vi "CTRE_Phoenix_MotorControl_ConfigClosedLoopConstants.vi"(0 "CAN Talon SRX Ref":T1={"DeviceStatus"={"status"=FALSE, "code"=0, "source"=""}, "Type"=enum."PWM", "PWM"={"PWM Channel"=enum."PWM 1", "DeadBand"={"Name"="", "maxPositivePwm"=0, "minPositivePwm"=0, "centerPwm"=0, "maxNegativePwm"=0, "minNegativePwm"=0, "angularRange"=0}}, "CAN"={"Device Number"=0, "SetOutput VI Ref"=variant(enum8{"Percent VBus", "Current", "Speed", "Position", "Voltage"} enum."Percent VBus"), "GetOutput VI Ref"=variant(refnum<k1> refnum), "Enable VI Ref"=variant(dbl 12.0), "Disable VI Ref"=variant(enum8{"Percent VBus", "Speed", "Position", "Slave", "Unchanged / Invalid", "Voltage Compensation", "Current", "Motion Profile"} enum."Percent VBus"), "Data"=variant}, "Invert"=FALSE}, 1 "slotIdx":i32, 5 "P":sgl, 7 "I":sgl, 9 "D":sgl, 11 "error in (no error)":errorcluster, 12 "F":sgl, 13 "I Zone":sgl, 14 "timeoutMs":i32) -> (4 "CAN Talon SRX Ref":T1={"DeviceStatus"={"status"=FALSE, "code"=0, "source"=""}, "Type"=enum."PWM", "PWM"={"PWM Channel"=enum."PWM 1", "DeadBand"={"Name"="", "maxPositivePwm"=0, "minPositivePwm"=0, "centerPwm"=0, "maxNegativePwm"=0, "minNegativePwm"=0, "angularRange"=0}}, "CAN"={"Device Number"=0, "SetOutput VI Ref"=variant(enum8{"Percent VBus", "Current", "Speed", "Position", "Voltage"} enum."Percent VBus"), "GetOutput VI Ref"=variant(refnum<k1> refnum), "Enable VI Ref"=variant(dbl 12.0), "Disable VI Ref"=variant(enum8{"Percent VBus", "Speed", "Position", "Slave", "Unchanged / Invalid", "Voltage Compensation", "Current", "Motion Profile"} enum."Percent VBus"), "Data"=variant}, "Invert"=FALSE}, 15 "error out":errorcluster)   [LabVIEW 2016]
doc: "Configures the closed-loop constant values."
uses:
  <vilib>/Rock Robotics/WPI/MotorControl/WPI_MotorControlDeviceRef.ctl
  <vilib>/Rock Robotics/WPI/MotorControl/WPI_MotorControlType.ctl
  <vilib>/Rock Robotics/SystemInterfaces/DIO/FPGA_DIOPWMChannel.ctl
  <vilib>/Rock Robotics/WPI/PWM/WPI_PWMDeadband.ctl
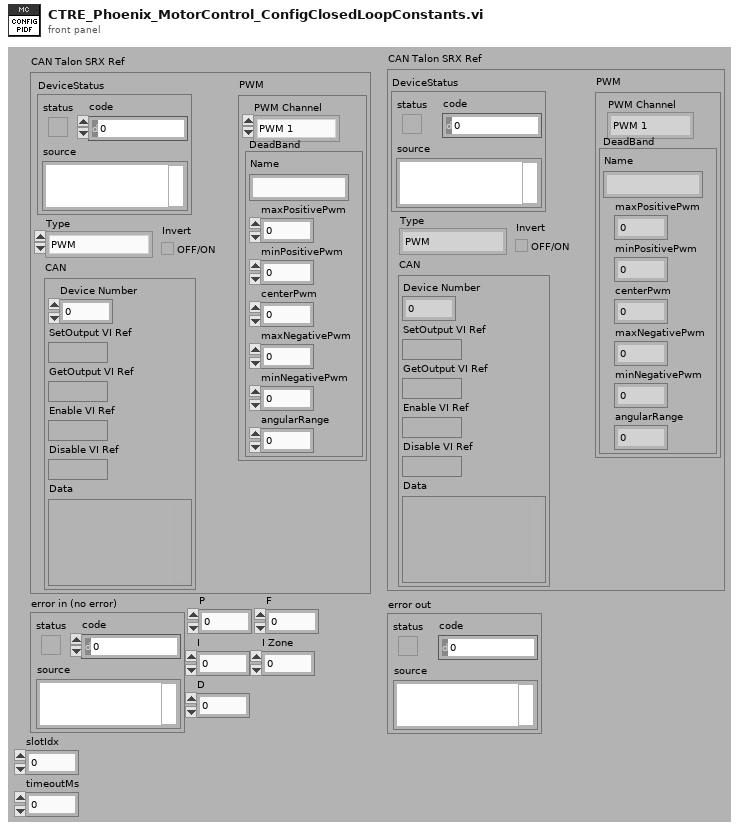
[diagram p1: front panel]
types:
  T1 = typedef "WPI_MotorControlDeviceRef.ctl" = cluster{"DeviceStatus":errorcluster, "Type":T2, "PWM":cluster{"PWM Channel":T3, "DeadBand":T4}, "CAN":cluster{"Device Number":u8, "SetOutput VI Ref":variant, "GetOutput VI Ref":variant, "Enable VI Ref":variant, "Disable VI Ref":variant, "Data":variant}, "Invert":bool}
  T2 = typedef "WPI_MotorControlType.ctl" = enum16{"PWM", "CAN"}
  T3 = typedef "FPGA_DIOPWMChannel.ctl" = enum8{"PWM 0", "PWM 1", "PWM 2", "PWM 3", "PWM 4", "PWM 5", "PWM 6", "PWM 7", "PWM 8", "PWM 9", "PWM MXP 0", "PWM MXP 1", "PWM MXP 2", "PWM MXP 3", "PWM MXP 4", "PWM MXP 5", "PWM MXP 6", "PWM MXP 7", "PWM MXP 8", "PWM MXP 9", "Invalid"}
  T4 = typedef "WPI_PWMDeadband.ctl" = cluster{"Name":string, "maxPositivePwm":i32, "minPositivePwm":i32, "centerPwm":i32, "maxNegativePwm":i32, "minNegativePwm":i32, "angularRange":u16}
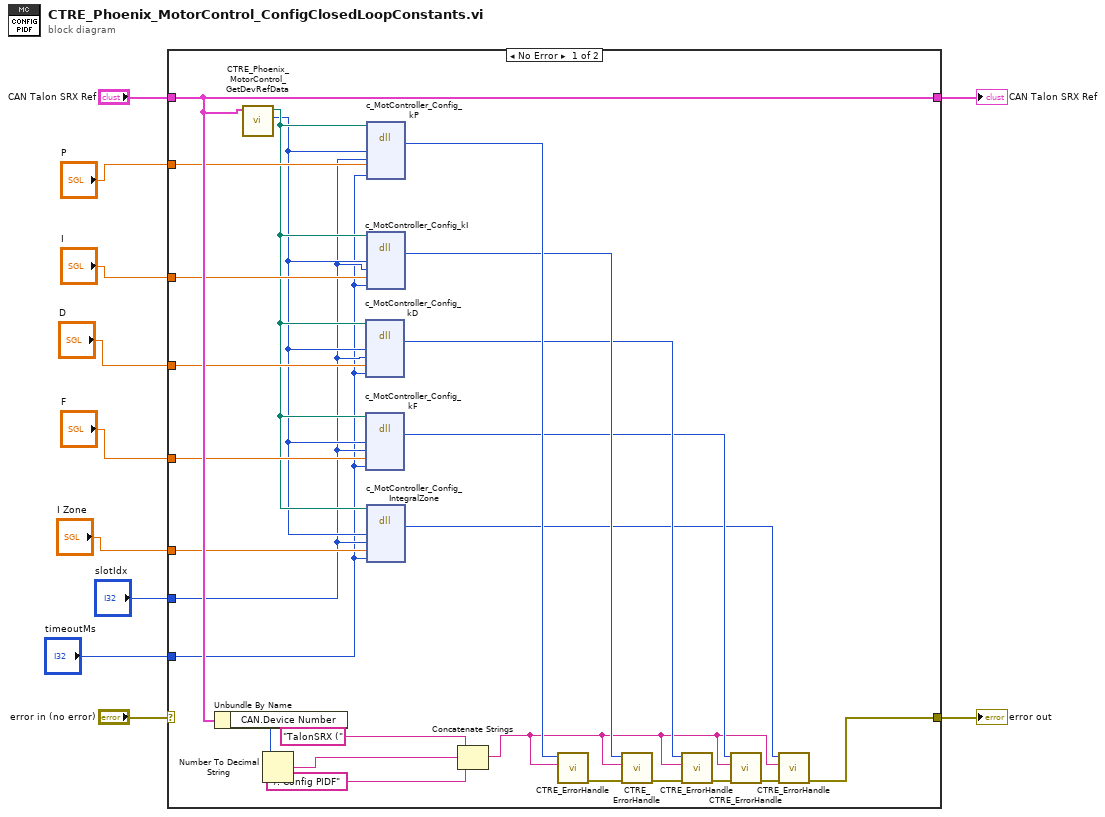
[diagram p0: block diagram]
diagram:
  n1 = case shown="No Error" "error in (no error)" {
    selector: "error in (no error)" -> [_ w38]
    tunnel: [w14 w38] -> w11
    tunnel: "CAN Talon SRX Ref" -> [w32 w37]
    tunnel: [w32 w37] -> w9
    tunnel: "P" -> [w29 _]
    tunnel: "I" -> [w28 _]
    tunnel: "D" -> [w27 _]
    tunnel: "F" -> [w26 _]
    tunnel: "I Zone" -> [w25 _]
    tunnel: "slotIdx" -> [w13 _]
    tunnel: "timeoutMs" -> [w12 _]
    frame No Error {
      n2 = Unbundle By Name(w32) -> ("CAN.Device Number"=w33:u8)
      n3 = call "CTRE_Phoenix_MotorControl_GetDevRefData.vi"("MotorControlDevRef"=w32) -> ("handle"=w23:u64, "Library"=w24:path)  [unwired: 4 in, 5 out]
      n4 = Number To Decimal String(number=w33) -> (decimal integer string=w35:string)  [unwired: 1 in]
      n5 = dll-call lib="?" fn="c_MotController_Config_kD"(path in=w24, "handle"=w23, "slotIdx"=w13, "value"=w27, "timeoutMs"=w12) -> ("ErrorCode"=w20:i32)  [unwired: 6 in, 2 out]
      n6 = dll-call lib="?" fn="c_MotController_Config_kF"(path in=w24, "handle"=w23, "slotIdx"=w13, "value"=w26, "timeoutMs"=w12) -> ("ErrorCode"=w18:i32)  [unwired: 6 in, 2 out]
      n7 = dll-call lib="?" fn="c_MotController_Config_kP"(path in=w24, "handle"=w23, "slotIdx"=w13, "value"=w29, "timeoutMs"=w12) -> ("ErrorCode"=w31:i32)  [unwired: 6 in, 2 out]
      n8 = dll-call lib="?" fn="c_MotController_Config_kI"(path in=w24, "handle"=w23, "slotIdx"=w13, "value"=w28, "timeoutMs"=w12) -> ("ErrorCode"=w22:i32)  [unwired: 6 in, 2 out]
      n9 = dll-call lib="?" fn="c_MotController_Config_IntegralZone"(path in=w24, "handle"=w23, "slotIdx"=w13, "value"=w25, "timeoutMs"=w12) -> ("ErrorCode"=w15:i32)  [unwired: 6 in, 2 out]
      n10 = Concatenate Strings("TalonSRX (" ("string"), w35, "): Config PIDF" ("string")) -> (w16:string)
      n11 = call "CTRE_ErrorHandle.vi"("origin"=w16, "code"=w31) -> ("error out"=w30:errorcluster)  [unwired: 9 in]
      n12 = call "CTRE_ErrorHandle.vi"("error in"=w30, "origin"=w16, "code"=w22) -> ("error out"=w21:errorcluster)  [unwired: 8 in]
      n13 = call "CTRE_ErrorHandle.vi"("error in"=w21, "origin"=w16, "code"=w20) -> ("error out"=w19:errorcluster)  [unwired: 8 in]
      n14 = call "CTRE_ErrorHandle.vi"("error in"=w19, "origin"=w16, "code"=w18) -> ("error out"=w17:errorcluster)  [unwired: 8 in]
      n15 = call "CTRE_ErrorHandle.vi"("error in"=w17, "origin"=w16, "code"=w15) -> ("error out"=w14:errorcluster)  [unwired: 8 in]
    }
    frame Error {
    }
  }
  "CAN Talon SRX Ref" <- w9
  "error out" <- w11
